vi "Build Path Multi-OS.vi"(1 "name or relative path":string, 2 "base path":path) -> (0 "appended path":path)   [LabVIEW 2021, in "File_CIF_U.lvlib"]
doc: "The Build Path does not automatically handle OS specific file path elements of / and \\. This adjusts so the same code will work on Linux and Windows targets."
uses:
  File_CIF_U.lvlib
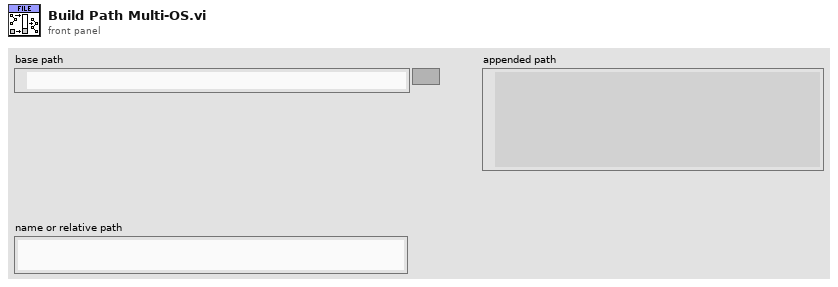
[diagram p1: front panel]
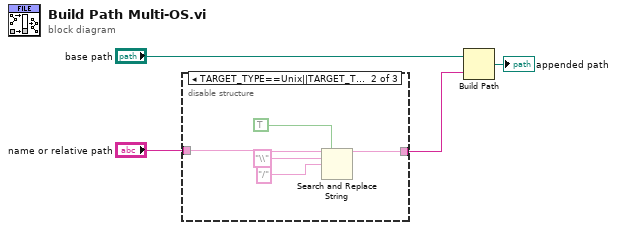
[diagram p0: block diagram]
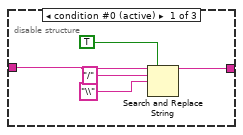
[diagram p2: hidden frame]
diagram:
  n1 = disable-structure shown="TARGET_TYPE==Unix||TARGET_TYPE==RT" {
    disable-tunnel: "name or relative path" -> [w9 w14 w15]
    disable-tunnel: [w5 w10 w15] -> w2
    frame condition #0 (active) {
      n2 = Search and Replace String(replace all?=TRUE ("replace all? (F)"), input string=w9, search string="/", replace string="\\" ("replace string (\"\")")) -> (result string=w5:string)  [unwired: 4 in, 3 out]
    }
    frame condition #1 {
      n3 = Search and Replace String(replace all?=TRUE ("replace all? (F)"), input string=w14, search string="\\", replace string="/" ("replace string (\"\")")) -> (result string=w10:string)  [unwired: 4 in, 3 out]
    }
    frame condition #2 {
    }
  }
  n4 = Build Path(base path="base path", name or relative path=w2) -> (appended path=→"appended path":path)
